vi "Generate Response Head.vi"(9 "Value":string, 10 "Header":string(combo)="User-Agent" caption="文件头", 11 "HEADIN":string) -> (3 "HEADOUT":string)   [LabVIEW 2019, in "HTTP Server.lvlib"]
uses:
  HTTP Server.lvlib
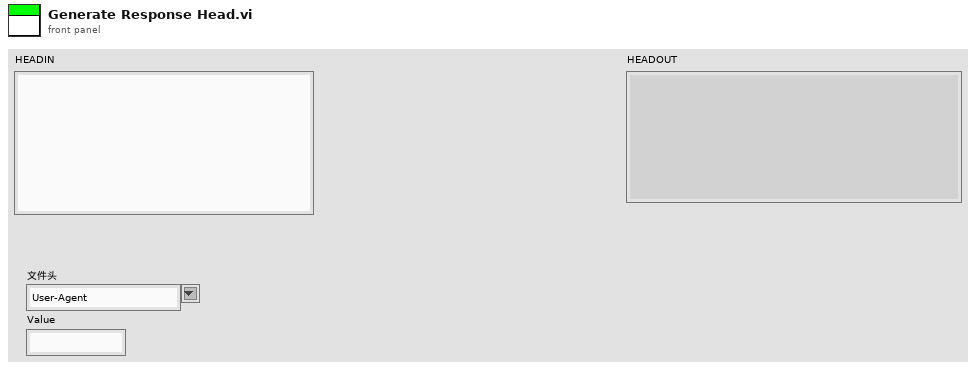
[diagram p1: front panel]
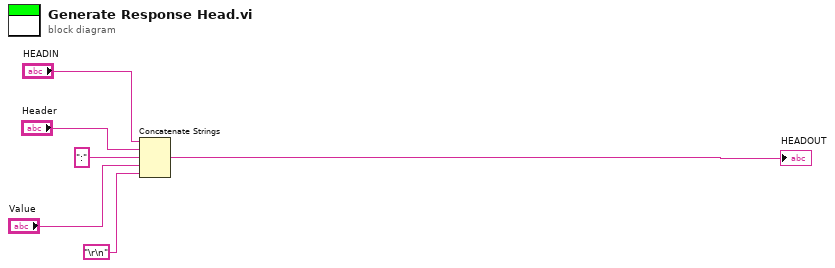
[diagram p0: block diagram]
diagram:
  n1 = Concatenate Strings("HEADIN", "Header", ":" ("字符串"), "Value", "\r\n") -> (→"HEADOUT":string)
